vi "H5Aget_type.vi"(6 "error in (no error)":errorcluster, 9 "HDF5 Attr Ref":T1) -> (0 "error out":errorcluster, 2 "HDF5 Datatype Ref":T1, 3 "HDF5 Attr Ref out":T1)   [LabVIEW 2017]
doc: "Gets an attribute datatype."
uses:
  <vilib>/UPVI/lvhdf5/library.llb/HDF5 Ref.ctl
  <vilib>/UPVI/lvhdf5/hdf5.dll
panel:
  # "LVHDF5 Toolkit\nCopyright (c) 2005-2013 by Jason D. Sommerville\nCopyright (c) 2014 by UPVI, LLC.\n\nThis use and distribution of this file is governed by the terms found in \nLICENSE.txt distributed with this toolkit and installed at\n <user.lib>\\_lvhdf5\\LICENSE.txt"
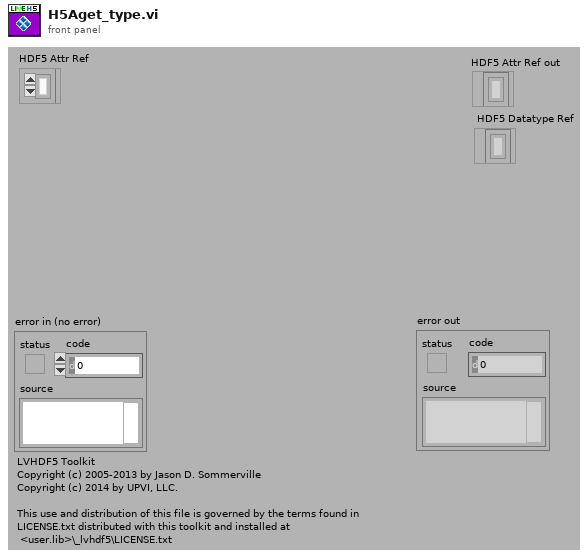
[diagram p1: front panel]
types:
  T1 = typedef "HDF5 Ref.ctl" = refnum<k1>
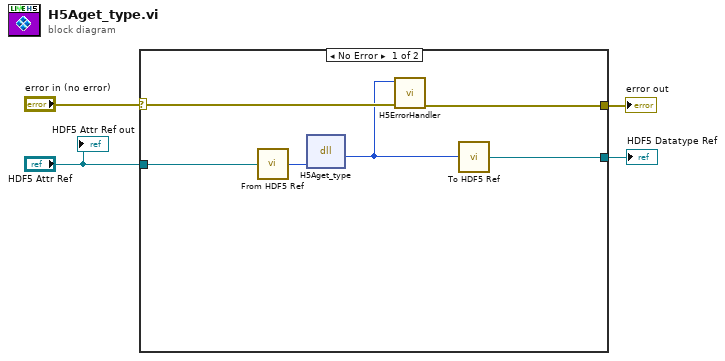
[diagram p0: block diagram]
diagram:
  n1 = case shown="No Error" "error in (no error)" {
    selector: "error in (no error)" -> [w8 w11]
    tunnel: [w5 w11] -> w2
    tunnel: "HDF5 Attr Ref" -> [w10 _]
    tunnel: [w6 _] -> w1
    frame No Error {
      n2 = call <vilib>:"From HDF5 Ref.vi"("HDF5 Ref"=w10) -> ("I32"=w9:i32)
      n3 = dll-call lib="C:/Program Files/National Instruments/LabVIEW 2017/vi.lib/UPVI/lvhdf5/hdf5.dll" fn="H5Aget_type"("attr_id"=w9) -> ("return type"=w7:i32)  [unwired: 4 in, 2 out]
      n4 = call <vilib>:"H5ErrorHandler.vi"("error in (no error)"=w8, "herr_t"=w7) -> ("error out"=w5:errorcluster)  [unwired: 3 in, 4 out]
      n5 = call <vilib>:"To HDF5 Ref.vi"("I32"=w7) -> ("HDF5 Ref"=w6:T1)
    }
    frame Error {
    }
  }
  "error out" <- w2
  "HDF5 Datatype Ref" <- w1
  "HDF5 Attr Ref out" <- "HDF5 Attr Ref"
